vi "String Array to String with Commas.vi"(1 "Array":string[](array[string])) -> (0 "String":string)   [LabVIEW 2019, in "LV-Data.PGSQL.lvclass"]
uses:
  LV-Data.PGSQL.lvclass
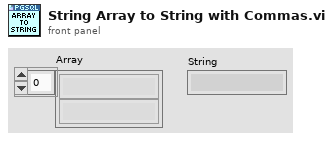
[diagram p1: front panel]
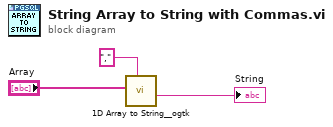
[diagram p0: block diagram]
diagram:
  n1 = call <userlib>:"1D Array to String__ogtk.vi"("delimiter (Tab)"="," ("string"), "Array of Strings"="Array") -> ("delimited string"=→"String":string)  [unwired: 9 in]
